vi "to_u16.vi"(8 "error in (no error)":errorcluster, 11 "U16 in":refnum<class "U16.lvclass">) -> (0 "error out":errorcluster, 3 "u16":u16)   [LabVIEW 2020, in "variant.lvlib" / "U16.lvclass"]
uses:
  U16.lvclass
  C:/projects/OpenG-Variant-Data-Library/source/library/Bytes/Bytes.lvclass
  Bytes/Bytes.lvclass/Bytes.ctl
  Bytes/Bytes.lvclass
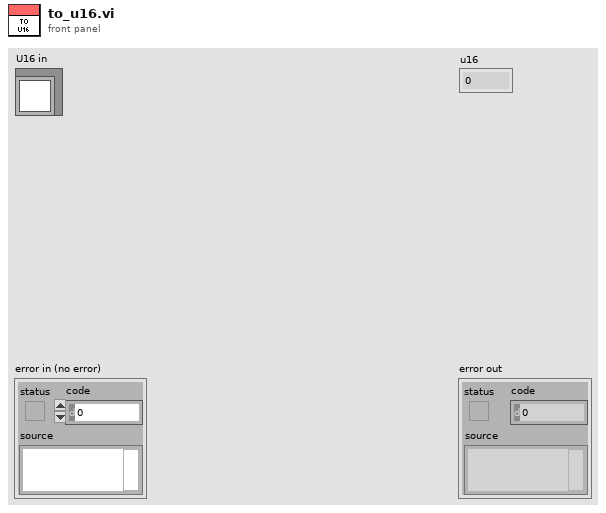
[diagram p1: front panel]
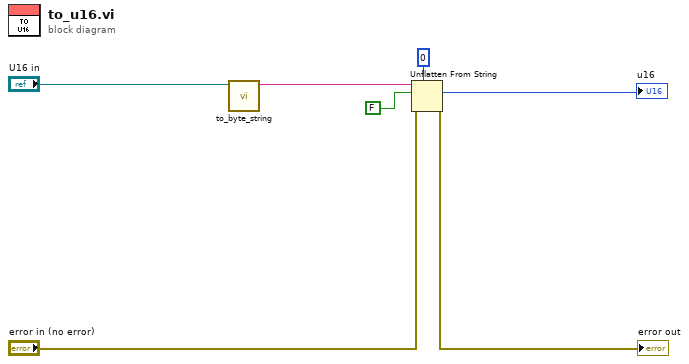
[diagram p0: block diagram]
diagram:
  n1 = call "to_byte_string.vi"("Bytes in"="U16 in") -> ("byte string"=w6:string)  [unwired: 10 in]
  n2 = Unflatten From String(type=u16 0 ("length"), binary string=w6, data includes array or string size? (T)=FALSE, error in (no error)="error in (no error)") -> (value=→"u16":u16, error out=→"error out":errorcluster)  [unwired: 1 in, 1 out]
